vi "Frame Update Data From UI Ref.vi"(8 "error in (no error)":errorcluster, 11 "IDE simple in":refnum<class "Main Panel.lvclass">) -> (0 "error out":errorcluster, 3 "IDE simple out":refnum<class "Main Panel.lvclass">)   [LabVIEW 2018, in "Main Panel.lvlib" / "Main Panel.lvclass"]
uses:
  Main Panel.lvclass
  Main Panel.lvclass/Main Panel.ctl
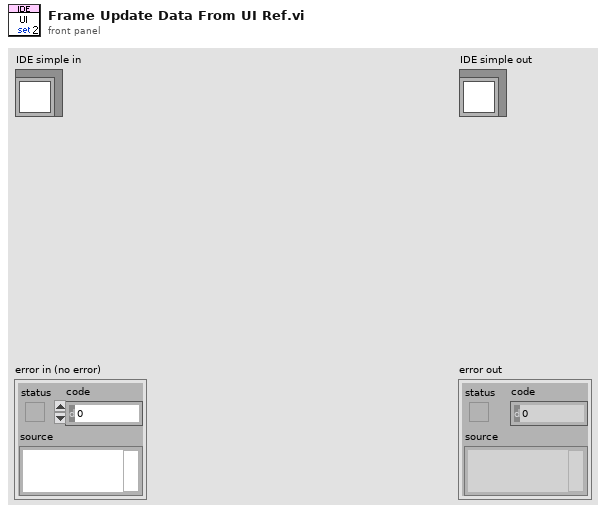
[diagram p1: front panel]
types:
  T1 = typedef "Data Parser.lvclass/frame b data.ctl" = cluster{"kind":string, "x":string, "y":string, "w":string, "h":string}
  T2 = typedef "Data Parser.lvclass/frame i data.ctl" = cluster{"kind":string, "x":string, "y":string, "w":string, "h":string, "dvx":string, "dvy":string, "dvz":string, "fall":string, "arest":string, "vrest":string, "bdefend":string, "injury":string, "zwidth":string, "effect":string, "catchingact":string, "caughtact":string}
  T3 = typedef "Data Parser.lvclass/frame title.ctl" = cluster{"Number":string, "Name":string}
  T4 = typedef "Data Parser.lvclass/frame basic data.ctl" = cluster{"Basic":cluster{"pic":string, "state":string, "wait":string, "next":string}, "Move":cluster{"dvx":string, "dvy":string, "dvz":string}, "Pic Center":cluster{"centerx":string, "centery":string}, "Skill":cluster{"hit_a":string, "hit_d":string, "hit_j":string, "hit_Fa":string, "hit_Ua":string, "hit_Da":string, "hit_Fj":string, "hit_Uj":string, "hit_Dj":string, "hit_ja":string}, "Mp":string}
  T5 = typedef "Data Parser.lvclass/frame o data.ctl" = cluster{"kind":string, "x":string, "y":string, "action":string, "dvx":string, "dvy":string, "dvz":string, "oid":string, "facing":string}
  T6 = typedef "Data Parser.lvclass/frame bp data.ctl" = cluster{"x":string, "y":string}
  T7 = typedef "Data Parser.lvclass/frame c data.ctl" = cluster{"kind":string, "x":string, "y":string, "injury":string, "cover":string, "vaction":string, "aaction":string, "taction":string, "hurtable":string, "decrease":string, "fronthurtact":string, "backhurtact":string, "dircontrol":string, "throwvx":string, "throwvy":string, "throwvz":string, "throwinjury":string}
  T8 = typedef "Data Parser.lvclass/frame w data.ctl" = cluster{"kind":string, "x":string, "y":string, "weaponact":string, "dvx":string, "dvy":string, "dvz":string, "attacking":string, "cover":string}
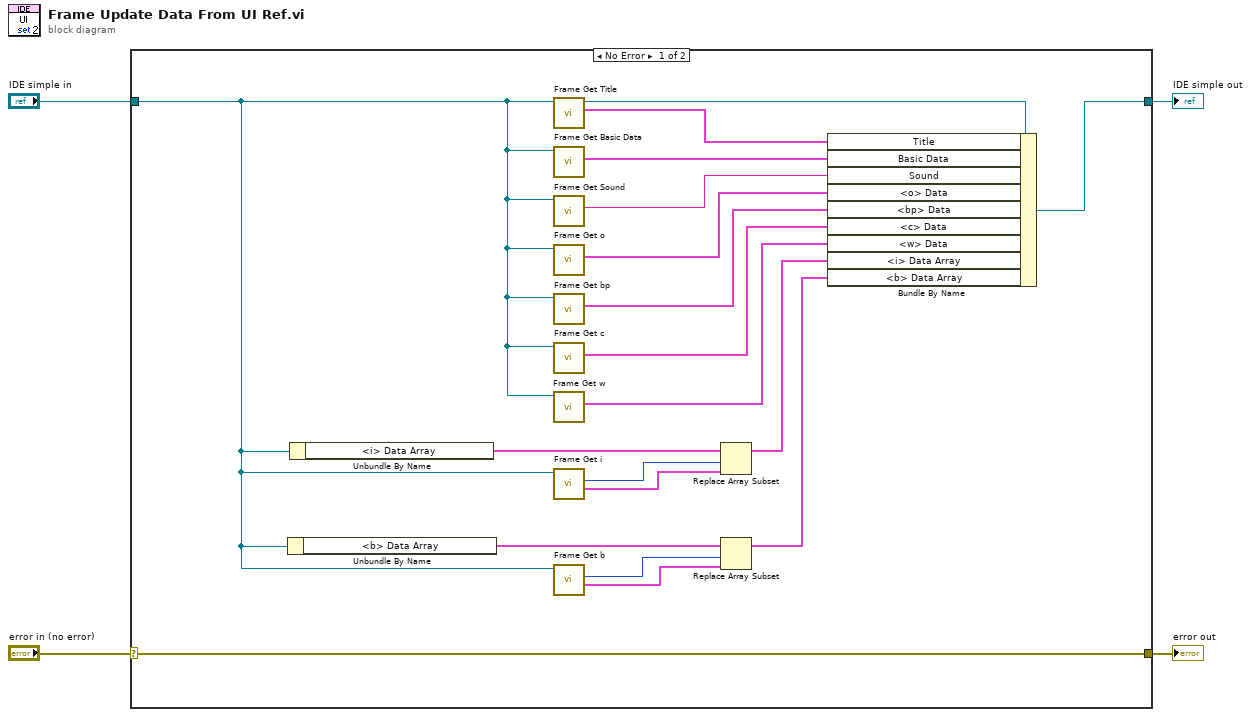
[diagram p0: block diagram]
diagram:
  n1 = case shown="No Error" "error in (no error)" {
    selector: "error in (no error)" -> [w6 w25]
    tunnel: [w6 w25] -> w3
    tunnel: [w7 w24] -> w1
    tunnel: "IDE simple in" -> [w5 w24]
    frame No Error {
      n2 = Unbundle By Name(w5) -> ("<b> Data Array"=w12:T1[])
      n3 = Unbundle By Name(w5) -> ("<i> Data Array"=w15:T2[])
      n4 = call "Frame Get Title.vi"("IDE simple in"=w5) -> ("Frame Title"=w22:T3, "IDE simple out"=w23:refnum<class "Main Panel.lvclass">)  [unwired: 8 in, 1 out]
      n5 = call "Frame Get Basic Data.vi"("IDE simple in"=w5) -> ("Frame Basic Data"=w21:T4)  [unwired: 8 in, 2 out]
      n6 = call "Frame Get Sound.vi"("IDE simple in"=w5) -> ("Sound String"=w20:string)  [unwired: 8 in, 2 out]
      n7 = call "Frame Get o.vi"("IDE simple in"=w5) -> ("<o> Data"=w19:T5)  [unwired: 8 in, 2 out]
      n8 = call "Frame Get bp.vi"("IDE simple in"=w5) -> ("<bp> Data"=w18:T6)  [unwired: 8 in, 2 out]
      n9 = call "Frame Get c.vi"("IDE simple in"=w5) -> ("<c> Data"=w17:T7)  [unwired: 8 in, 2 out]
      n10 = call "Frame Get w.vi"("IDE simple in"=w5) -> ("<w> Data"=w16:T8)  [unwired: 8 in, 2 out]
      n11 = call "Frame Get i.vi"("IDE simple in"=w5) -> ("<i> Data"=w13:T2, "Iindex"=w14:u32)  [unwired: 7 in, 2 out]
      n12 = call "Frame Get b.vi"("IDE simple in"=w5) -> ("<b> Data"=w10:T1, "Index"=w11:u32)  [unwired: 7 in, 2 out]
      n13 = Replace Array Subset(array=w15, new element=w13, index=w14) -> (w9:T2[])
      n14 = Replace Array Subset(array=w12, new element=w10, index=w11) -> (w8:T1[])
      n15 = Bundle By Name(cluster=w23, "Title"=w22, "Basic Data"=w21, "Sound"=w20, "<o> Data"=w19, "<bp> Data"=w18, "<c> Data"=w17, "<w> Data"=w16, "<i> Data Array"=w9, "<b> Data Array"=w8) -> (w7:refnum<class "Main Panel.lvclass">)
    }
    frame Error {
    }
  }
  "error out" <- w3
  "IDE simple out" <- w1
